vi "显示曲线.vi"() -> (0 "曲线数组":cluster{i32[], sgl[]}[](array[cluster]))   [LabVIEW 2018]
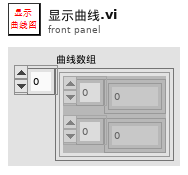
[diagram p1: front panel]
types:
  T1 = cluster{"Fx":sgl[], "Fy":sgl[], "Dx":sgl[], "Dy":sgl[]}
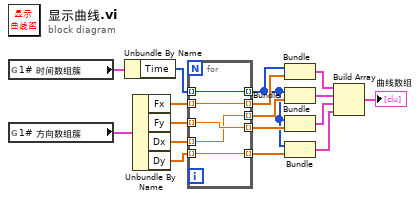
[diagram p0: block diagram]
diagram:
  n1 = global read "全局 1.vi" "1# 时间数组簇"() -> (w16:cluster{"Time":i32[]})
  n2 = global read "全局 1.vi" "1# 方向数组簇"() -> (w17:T1)
  n3 = Unbundle By Name(w16) -> ("Time"=w14:i32[])
  n4 = Unbundle By Name(w17) -> ("Fx"=w15:sgl[], "Fy"=w13:sgl[], "Dx"=w12:sgl[], "Dy"=w11:sgl[])
  n5 = for {
    tunnel: w15 -> [w22] mode=indexing
    tunnel: w14 -> [w21] mode=indexing
    tunnel: [w22] -> w10 mode=indexing
    tunnel: [w21] -> w4 mode=indexing
    tunnel: [w20] -> w6 mode=indexing
    tunnel: w13 -> [w20] mode=indexing
    tunnel: [w19] -> w8 mode=indexing
    tunnel: w12 -> [w19] mode=indexing
    tunnel: [w18] -> w3 mode=indexing
    tunnel: w11 -> [w18] mode=indexing
  }
  n6 = Bundle(w4, w10) -> (w9:cluster{i32[], sgl[]})  [unwired: 1 in]
  n7 = Bundle(w4, w8) -> (w7:cluster{i32[], sgl[]})  [unwired: 1 in]
  n8 = Bundle(w4, w6) -> (w5:cluster{i32[], sgl[]})  [unwired: 1 in]
  n9 = Bundle(w4, w3) -> (w2:cluster{i32[], sgl[]})  [unwired: 1 in]
  n10 = Build Array(w9, w7, w5, w2) -> (→"曲线数组":cluster{i32[], sgl[]}[])
